vi "Entity Template Path.vi"() -> (2 "New Entity Template":path)   [LabVIEW 2020, in "Conditu2.lvlib"]
uses:
  Conditu2.lvlib
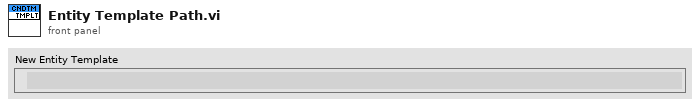
[diagram p1: front panel]
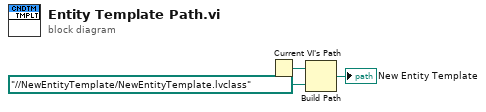
[diagram p0: block diagram]
diagram:
  n1 = Current VI's Path() -> (path=w3:path)
  n2 = Build Path(base path=w3, name or relative path=path "../../NewEntityTemplate/NewEntityTemplate.lvclass" ("Relative Path from 1 to 2")) -> (appended path=→"New Entity Template":path)
